vi "Simple F-70 controller.vi"() -> ()   [LabVIEW 2021, in "F-70 controller.lvlib"]
uses:
  F-70 controller.lvlib
  controls/F-70 controller states.ctl
  controls/F-70 controller commands.ctl
  controls/Message to F-70 controller.ctl
  controls/F-70 controller properties.ctl
  <instrlib>/F-70 driver/F-70 driver.lvlib
  <instrlib>/F-70 driver/public/F-70 parameters.ctl
panel:
  out "Event log":string[](array[string])
  in  "Search btn":bool
  out "F-70 parameters":T1 {"Last updated" format="%<%d/%m/%Y %H:%M:%S>T"; "State of operation" items=["Local Off", "Local On", "Remote Off", "Remote On", "Cold head Run", "Cold head pause", "Fault Off", "Oil Fault Off"]; "Return pressure (PSIG)" scale=0.0..200.0; "Water in Tmp (°C)" scale=0.0..100.0; "Water out Tmp (°C)" scale=0.0..100.0; "He discharge Tmp (°C)" scale=0.0..100.0}
  in  "Start Stop Cold head btn":bool
  in  "Exit app btn":bool
  in  "Update interval (ms)":i32=5000
  in  "error in (no error)":errorcluster
  out "error out":errorcluster
  in  "Start Stop btn":bool
  in  "Connect btn":bool
  in  "VISA resource name":refnum<visa-resource-name>
  # "Simple F-70 controller"
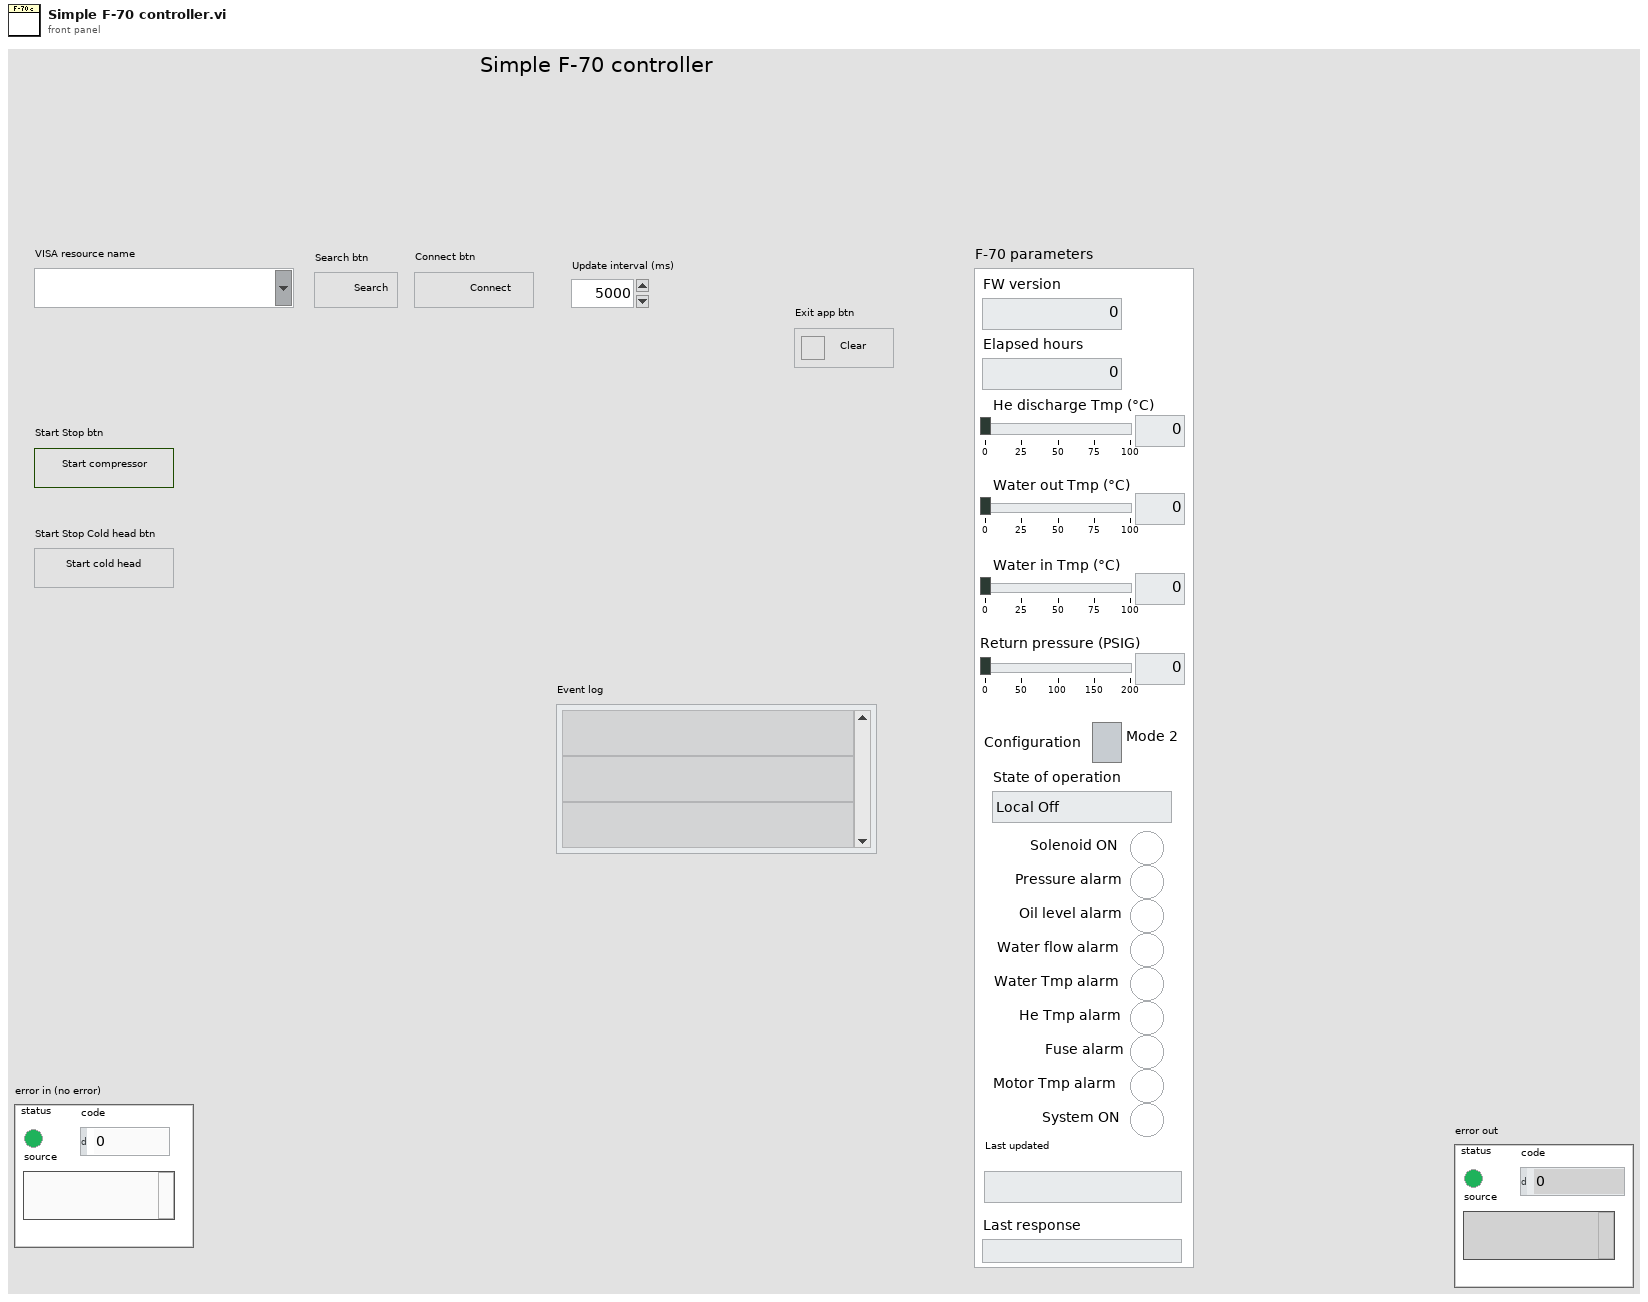
[diagram p1: front panel]
types:
  T1 = typedef "F-70 driver.lvlib/F-70 parameters.ctl" = cluster{"FW version":dbl, "Elapsed hours":dbl, "He discharge Tmp (°C)":dbl, "Water out Tmp (°C)":dbl, "Water in Tmp (°C)":dbl, "Return pressure (PSIG)":dbl, "Configuration":bool, "State of operation":u16, "Solenoid ON":bool, "Pressure alarm":bool, "Oil level alarm":bool, "Water flow alarm":bool, "Water Tmp alarm":bool, "He Tmp alarm":bool, "Fuse alarm":bool, "Motor Tmp alarm":bool, "System ON":bool, "Last updated":timestamp, "Last response":string}
  T2 = typedef "F-70 controller properties.ctl" = cluster{"Connected":bool, "Command msg":T3, "Data msg":variant, "Waiting msgs":i32, "Timeout counter":i32, "Logs":string[]}
  T3 = typedef "F-70 controller commands.ctl" = enum16{"Ignore", "Connect", "Read temperatures", "Read pressure", "Read status", "Update all", "Start compressor", "Stop compressor", "Clear error", "Disconnect"}
  T4 = typedef "F-70 controller.lvlib/F-70 controller states.ctl" = enum16{"Initialize GUI", "Wait for event", "Check message", "Execute command", "Send response", "Sleep", "Search device", "Reserved2", "End"}
  T5 = enum8{"Enabled", "Disabled", "Disabled and Grayed Out"}
  T6 = typedef "Message to F-70 controller.ctl" = cluster{"Command msg":T3, "Data msg":variant}
  T7 = enum16{"Left Button", "Center Button", "Right Button", "Window Close"}
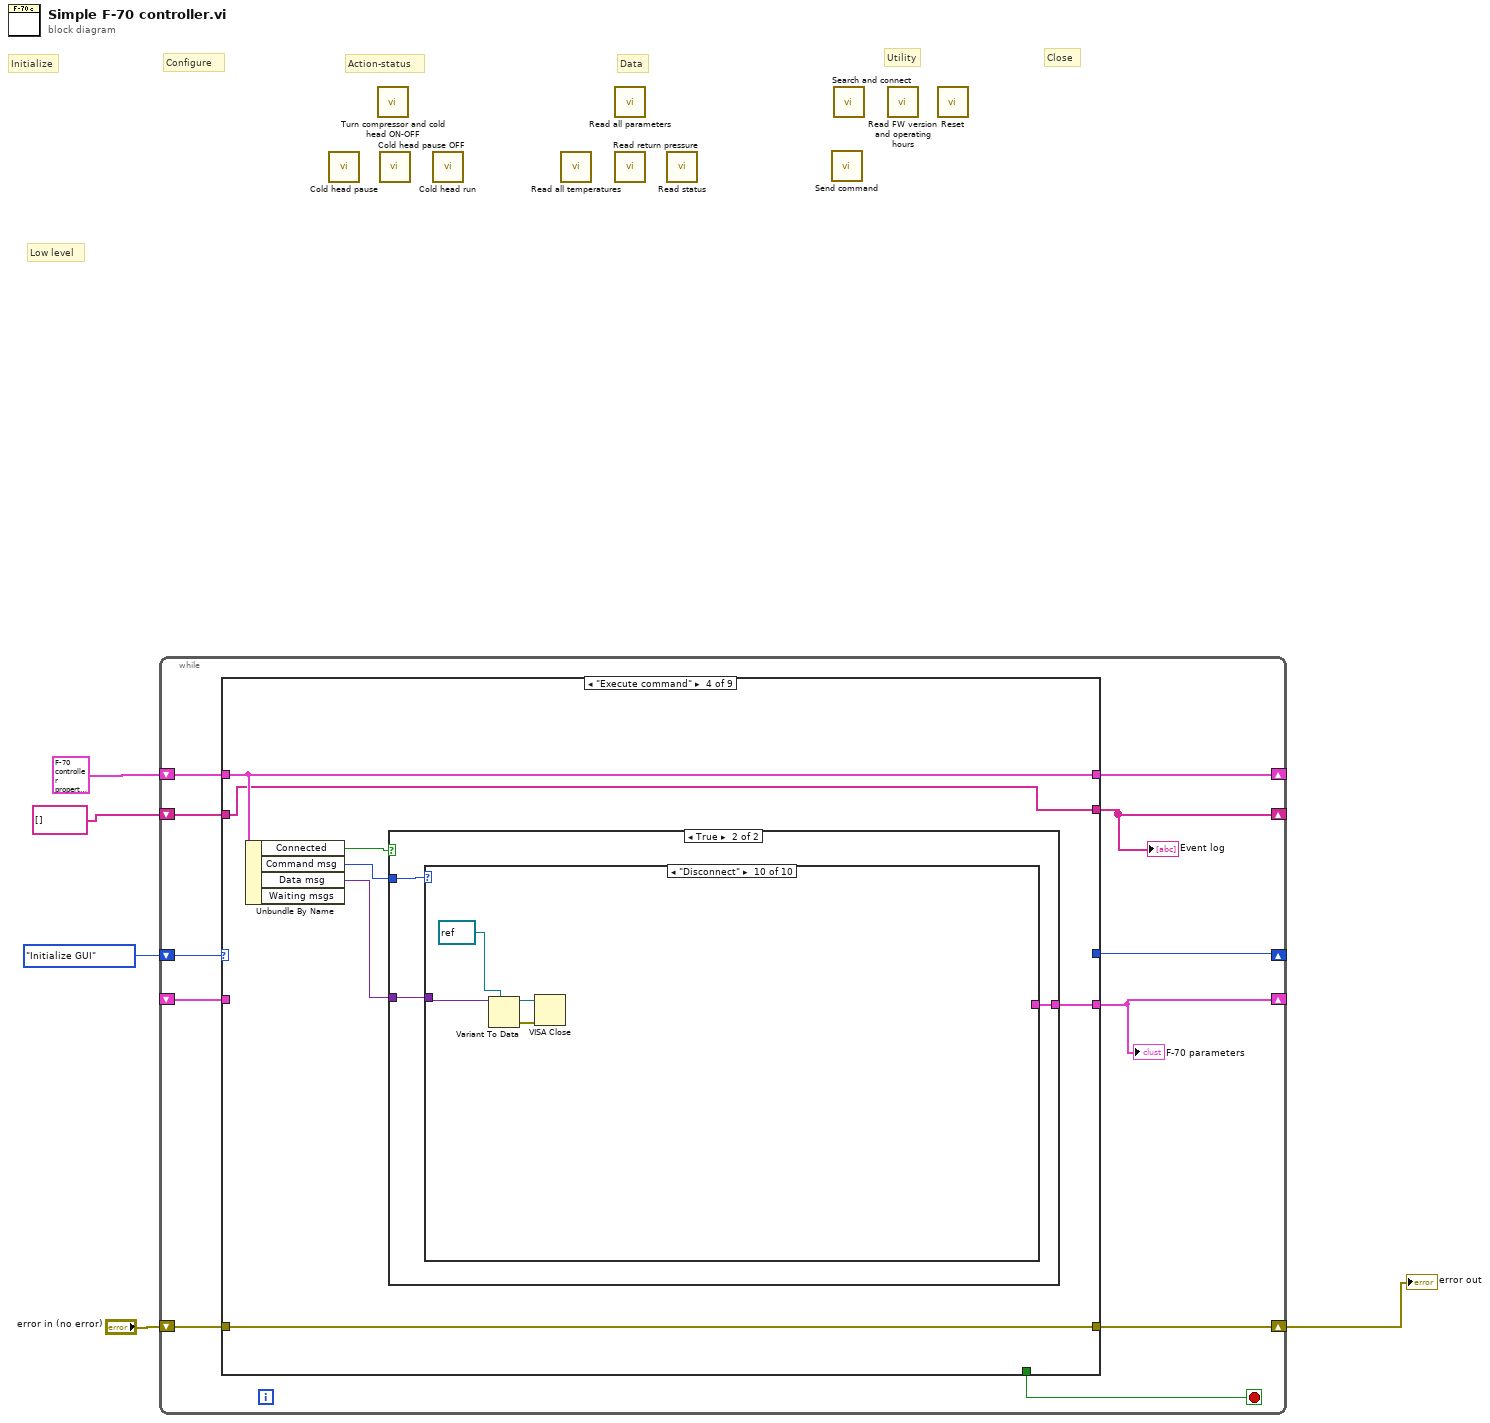
[diagram p0: block diagram]
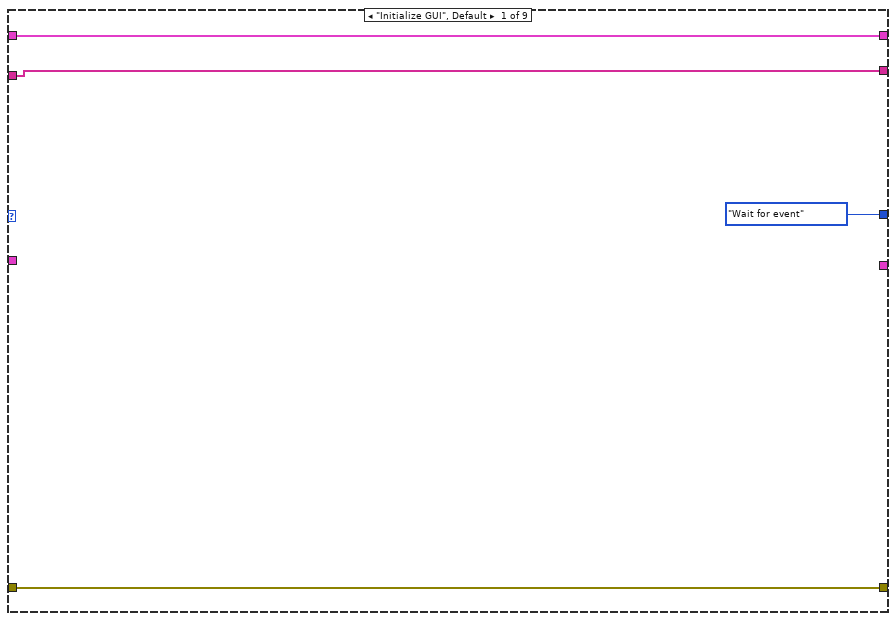
[diagram p2: hidden frame]
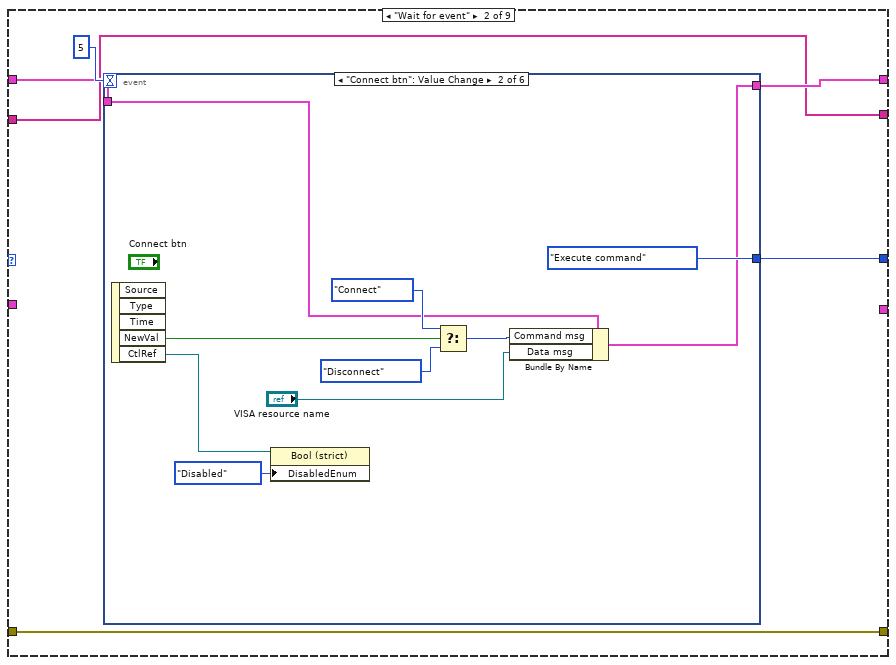
[diagram p3: hidden frame]
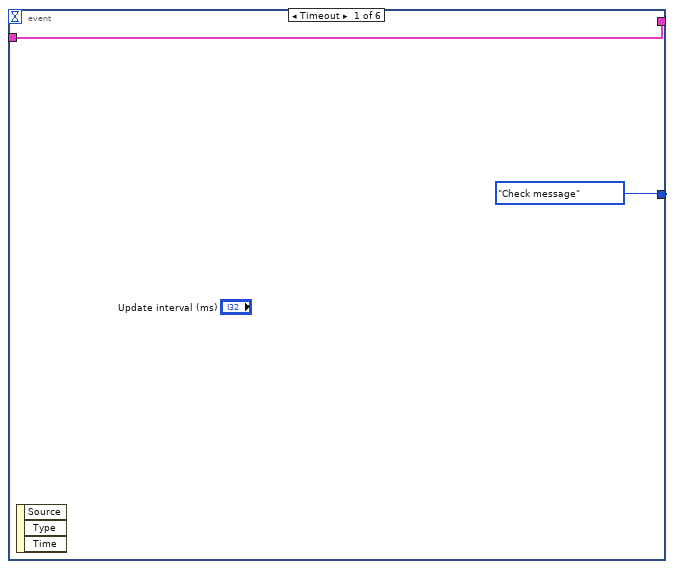
[diagram p4: hidden frame]
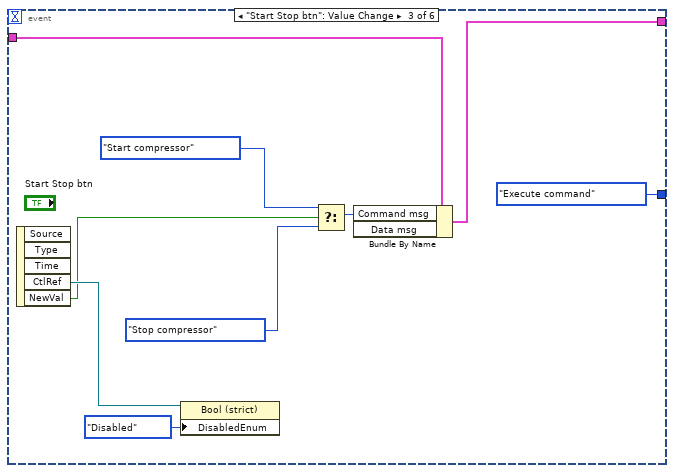
[diagram p5: hidden frame]
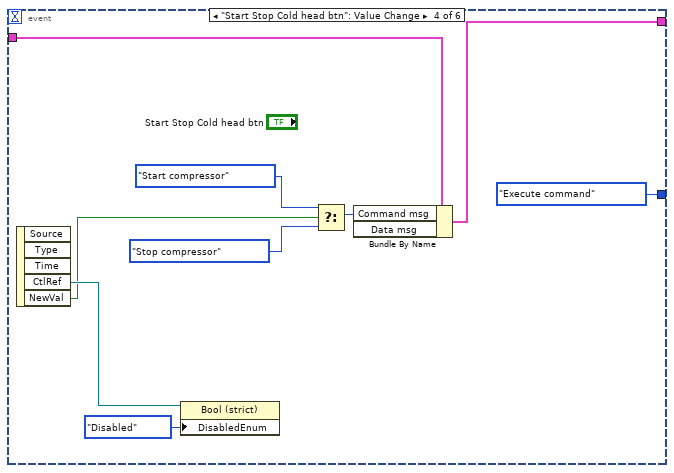
[diagram p6: hidden frame]
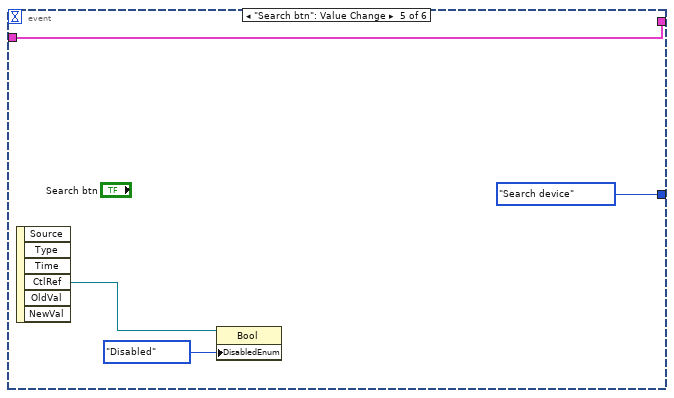
[diagram p7: hidden frame]
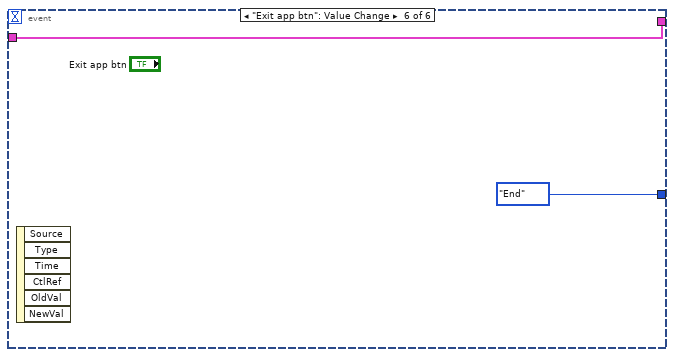
[diagram p8: hidden frame]
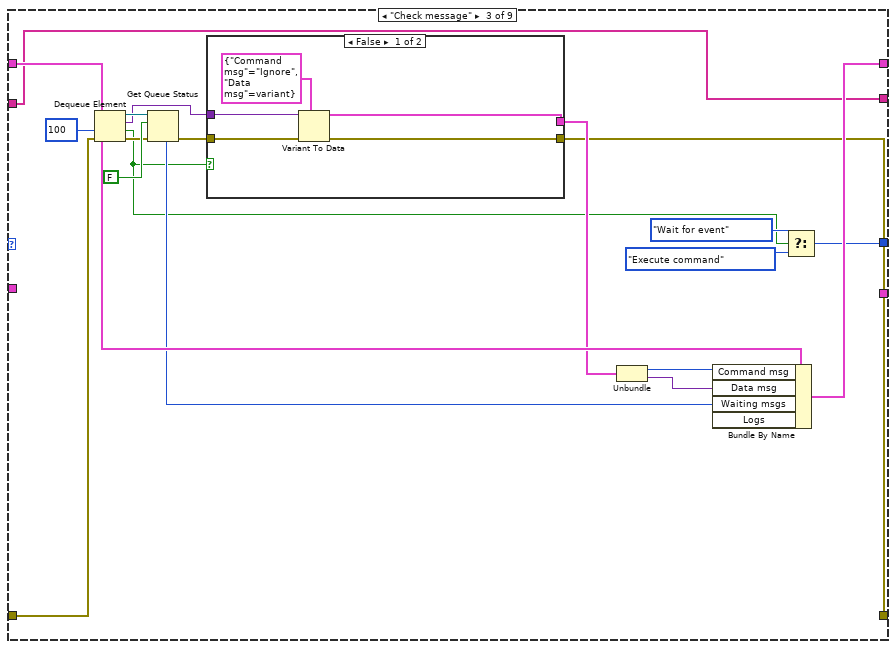
[diagram p9: hidden frame]
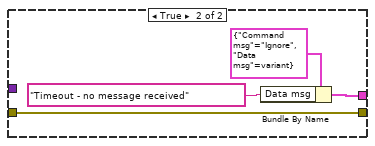
[diagram p10: hidden frame]
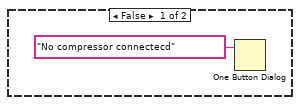
[diagram p11: hidden frame]
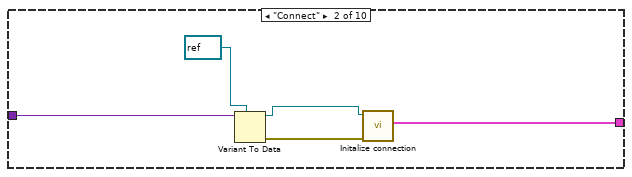
[diagram p13: hidden frame]
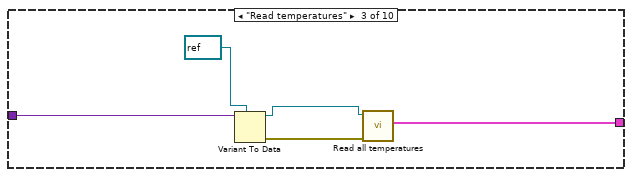
[diagram p14: hidden frame]
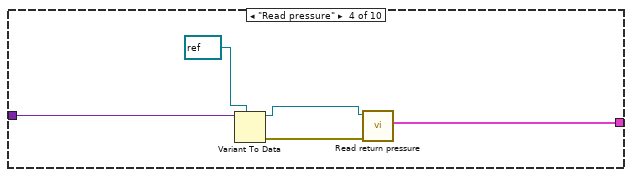
[diagram p15: hidden frame]
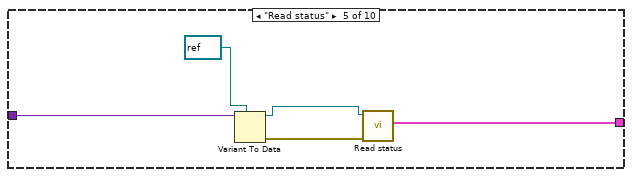
[diagram p16: hidden frame]
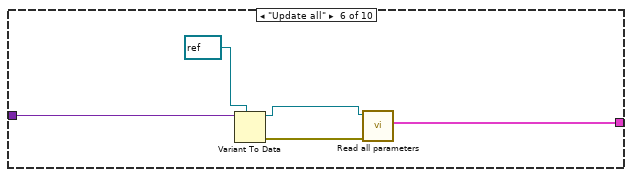
[diagram p17: hidden frame]
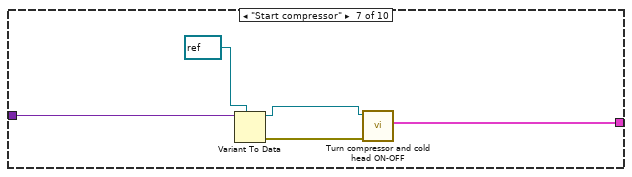
[diagram p18: hidden frame]
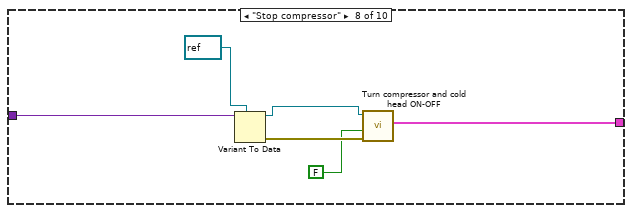
[diagram p19: hidden frame]
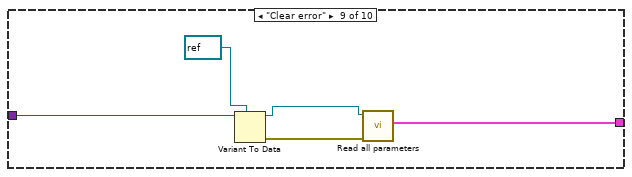
[diagram p20: hidden frame]
diagram:
  # "Low level"
  # "Action-status"
  # "Close"
  # "Utility"
  # "Data"
  # "Configure"
  # "Initialize"
  n1 = while {
    shift-right: [w15] -> _
    shift-left: F-70_controller_states."Initialize GUI" -> [w16]
    shift-right: [w13] -> _
    shift-left: T2 {"Connected"=FALSE, "Command msg"=enum."Ignore", "Data msg"=variant, "Waiting msgs"=0, "Timeout counter"=0, "Logs"=[]} ("F-70 controller properties") -> [w14]
    shift-right: [w11] -> w2
    shift-left: "error in (no error)" -> [w12]
    shift-right: [w10] -> _
    shift-left: string[] [] ("Event log") -> [w9]
    shift-right: [w7] -> _
    shift-left: _ -> [w6]
    stop <- w8 stop-if-true
    n2 = case shown="\"Execute command\"" w16 {
      tunnel: [F-70_controller_states."Wait for event" w25 w67 _ _ _ F-70_controller_states."Wait for event" ("f") _ w165] -> w15
      tunnel: w14 -> [w19 w24 w76 w96 w149 w152 w161 w164 w168]
      tunnel: [w19 w23 w70 w96 w149 w152 w161 w164 w168] -> w13
      tunnel: w12 -> [w18 w22 w77 w97 w148 w151 w160 w163 w170]
      tunnel: [w18 w22 w68 w97 w148 w151 w158 w163 w170] -> w11
      tunnel: w9 -> [w17 w21 w63 w95 w147 w150 w156 w162 w169]
      tunnel: [w17 w21 w63 w95 w147 w150 w156 w162 w169] -> w10
      tunnel: [_ _ _ _ _ _ _ _ w166] -> w8
      tunnel: [_ _ _ w91 _ _ _ _ _] -> w7
      tunnel: w6 -> [_ _ _ _ _ _ _ _ _]
      frame "Initialize GUI", Default {
      }
      frame "Wait for event" {
        n3 = event shown="[1] \"Connect btn\": Value Change" {
          selector: _ -> [_ _ _ _ _ _]
          dyn-events: _ -> [_ _ _ _ _ _]
          timeout: 5 -> [_ _ _ _ _ _]
          tunnel: [F-70_controller_states."Check message" F-70_controller_states."Execute command" F-70_controller_states."Execute command" F-70_controller_states."Execute command" F-70_controller_states."Search device" F-70_controller_states."End"] -> w25
          tunnel: w24 -> [w27 w32 w46 w55 w59 w61]
          tunnel: [w27 w37 w39 w48 w59 w61] -> w23
          event Timeout {
            n4 = event-data() -> ()  [unwired: 1 in, 3 out]
          }
          event "Connect btn": Value Change {
            n5 = event-data() -> ("NewVal"=w34:bool, "CtlRef"=w30:refnum<vi>)  [unwired: 1 in, 3 out]
            n6 = property class="Bool (strict)"(reference=w30, "DisabledEnum"=T5."Disabled" ("Disabled")) -> ()  [unwired: 1 in, 2 out]
            n7 = Select(t=F-70_controller_commands."Connect" ("Command msg"), s=w34, f=F-70_controller_commands."Disconnect") -> (s? t:f=w36:T3)
            n8 = Bundle By Name(cluster=w32, "Command msg"=w36, "Data msg"="VISA resource name") -> (w37:T2)
          }
          event "Start Stop btn": Value Change {
            n9 = event-data() -> ("CtlRef"=w44:refnum<vi>, "NewVal"=w41:bool)  [unwired: 1 in, 3 out]
            n10 = property class="Bool (strict)"(reference=w44, "DisabledEnum"=T5."Disabled" ("Disabled")) -> ()  [unwired: 1 in, 2 out]
            n11 = Select(t=F-70_controller_commands."Start compressor", s=w41, f=F-70_controller_commands."Stop compressor" ("Command msg")) -> (s? t:f=w45:T3)
            n12 = Bundle By Name(cluster=w46, "Command msg"=w45) -> (w39:T2)  [unwired: 1 in]
          }
          event "Start Stop Cold head btn": Value Change {
            n13 = event-data() -> ("CtlRef"=w53:refnum<vi>, "NewVal"=w50:bool)  [unwired: 1 in, 3 out]
            n14 = property class="Bool (strict)"(reference=w53, "DisabledEnum"=T5."Disabled" ("Disabled")) -> ()  [unwired: 1 in, 2 out]
            n15 = Select(t=F-70_controller_commands."Start compressor", s=w50, f=F-70_controller_commands."Stop compressor" ("Command msg")) -> (s? t:f=w54:T3)
            n16 = Bundle By Name(cluster=w55, "Command msg"=w54) -> (w48:T2)  [unwired: 1 in]
          }
          event "Search btn": Value Change {
            n17 = event-data() -> ("CtlRef"=w58:refnum<vi>)  [unwired: 1 in, 5 out]
            n18 = property class="Bool"(reference=w58, "DisabledEnum"=T5."Disabled" ("Disabled")) -> ()  [unwired: 1 in, 2 out]
          }
          event "Exit app btn": Value Change {
            n19 = event-data() -> ()  [unwired: 1 in, 6 out]
          }
        }
      }
      frame "Check message" {
        n20 = Dequeue Element(timeout in ms (-1)=100, error in (no error)=w77) -> (queue out=w78:refnum<queue>, element=w75:variant, timed out?=w65:bool, error out=w79:errorcluster)  [unwired: 1 in]
        n21 = Get Queue Status(queue=w78, return elements? (F)=FALSE, error in (no error)=w79) -> (error out=w74:errorcluster, # elements in queue=w69:i32)  [unwired: 6 out]
        n22 = case shown="False" w65 {
          tunnel: w75 -> [w86 _]
          tunnel: w74 -> [w84 w90]
          tunnel: [w83 w88] -> w73
          tunnel: [w82 w90] -> w68
          frame False {
            n23 = Variant To Data(error in=w84, type=T6 {"Command msg"=enum."Ignore", "Data msg"=variant}, Variant=w86) -> (data=w83:T6, error out=w82:errorcluster)
          }
          frame True {
            n24 = Bundle By Name(cluster=T6 {"Command msg"=enum."Ignore", "Data msg"=variant}, "Data msg"="Timeout - no message received") -> (w88:T6)
          }
        }
        n25 = Unbundle(w73) -> ("Command msg"=w71:T3, "Data msg"=w72:variant)
        n26 = Bundle By Name(cluster=w76, "Command msg"=w71, "Data msg"=w72, "Waiting msgs"=w69) -> (w70:T2)  [unwired: 1 in]
        n27 = Select(t=F-70_controller_states."Wait for event", s=w65, f=F-70_controller_states."Execute command") -> (s? t:f=w67:T4)
      }
      frame "Execute command" {
        n28 = Unbundle By Name(w96) -> ("Connected"=w94:bool, "Command msg"=w93:T3, "Data msg"=w92:variant)  [unwired: 1 out]
        n29 = case shown="True" w94 {
          tunnel: w93 -> [_ w101]
          tunnel: w92 -> [_ w100]
          tunnel: [_ w99] -> w91
          frame False {
            n30 = One Button Dialog(message="No compressor connectecd") -> ()  [unwired: 1 in, 1 out]
          }
          frame True {
            n31 = case shown="\"Disconnect\"" w101 {
              tunnel: w100 -> [_ w103 w108 w113 w118 w123 w128 w134 w139 w143]
              tunnel: [_ w102 w107 w112 w117 w122 w127 w133 w138 _] -> w99
              frame "Ignore", Default {
              }
              frame "Connect" {
                n32 = Variant To Data(type=refnum<visa-resource-name> refnum ("VISA resource name"), Variant=w103) -> (data=w105:refnum<visa-resource-name>, error out=w104:errorcluster)  [unwired: 1 in]
                n33 = call <instrlib>:"Initalize connection.vi"("error in (no error)"=w104, "VISA resource in"=w105) -> ("F-70 parameters out"=w102:T1)  [unwired: 3 in, 2 out]
              }
              frame "Read temperatures" {
                n34 = Variant To Data(type=refnum<visa-resource-name> refnum ("VISA resource name"), Variant=w108) -> (data=w110:refnum<visa-resource-name>, error out=w109:errorcluster)  [unwired: 1 in]
                n35 = call <instrlib>:"Read all temperatures.vi"("error in"=w109, "VISA resource in"=w110) -> ("F-70 parameters out"=w107:T1)  [unwired: 4 in, 5 out]
              }
              frame "Read pressure" {
                n36 = Variant To Data(type=refnum<visa-resource-name> refnum ("VISA resource name"), Variant=w113) -> (data=w115:refnum<visa-resource-name>, error out=w114:errorcluster)  [unwired: 1 in]
                n37 = call <instrlib>:"Read return pressure.vi"("error in"=w114, "VISA resource in"=w115) -> ("F-70 parameters out"=w112:T1)  [unwired: 2 in, 3 out]
              }
              frame "Read status" {
                n38 = Variant To Data(type=refnum<visa-resource-name> refnum ("VISA resource name"), Variant=w118) -> (data=w120:refnum<visa-resource-name>, error out=w119:errorcluster)  [unwired: 1 in]
                n39 = call <instrlib>:"Read status.vi"("error in"=w119, "VISA resource in"=w120) -> ("F-70 parameters out"=w117:T1)  [unwired: 2 in, 3 out]
              }
              frame "Update all" {
                n40 = Variant To Data(type=refnum<visa-resource-name> refnum ("VISA resource name"), Variant=w123) -> (data=w125:refnum<visa-resource-name>, error out=w124:errorcluster)  [unwired: 1 in]
                n41 = call <instrlib>:"Read all parameters.vi"("error in"=w124, "VISA resource in"=w125) -> ("F-70 parameters out"=w122:T1)  [unwired: 3 in, 2 out]
              }
              frame "Start compressor" {
                n42 = Variant To Data(type=refnum<visa-resource-name> refnum ("VISA resource name"), Variant=w128) -> (data=w130:refnum<visa-resource-name>, error out=w129:errorcluster)  [unwired: 1 in]
                n43 = call <instrlib>:"Turn compressor and cold head ON-OFF.vi"("error in"=w129, "VISA resource in"=w130) -> ("F-70 parameters out"=w127:T1)  [unwired: 6 in, 3 out]
              }
              frame "Stop compressor" {
                n44 = Variant To Data(type=refnum<visa-resource-name> refnum ("VISA resource name"), Variant=w134) -> (data=w136:refnum<visa-resource-name>, error out=w135:errorcluster)  [unwired: 1 in]
                n45 = call <instrlib>:"Turn compressor and cold head ON-OFF.vi"("error in"=w135, "Action (ON)"=FALSE, "VISA resource in"=w136) -> ("F-70 parameters out"=w133:T1)  [unwired: 5 in, 3 out]
              }
              frame "Clear error" {
                n46 = Variant To Data(type=refnum<visa-resource-name> refnum ("VISA resource name"), Variant=w139) -> (data=w141:refnum<visa-resource-name>, error out=w140:errorcluster)  [unwired: 1 in]
                n47 = call <instrlib>:"Read all parameters.vi"("error in"=w140, "VISA resource in"=w141) -> ("F-70 parameters out"=w138:T1)  [unwired: 3 in, 2 out]
              }
              frame "Disconnect" {
                n48 = Variant To Data(type=refnum<visa-resource-name> refnum ("VISA resource name"), Variant=w143) -> (data=w145:refnum<visa-resource-name>, error out=w144:errorcluster)  [unwired: 1 in]
                n49 = VISA Close(VISA resource name=w145, error in (no error)=w144) -> ()  [unwired: 1 out]
              }
            }
          }
        }
      }
      frame "Send response" {
      }
      frame "Sleep" {
      }
      frame "Search device" {
        n50 = call <instrlib>:"Search and connect.vi"("error in"=w160) -> ("error out"=w154:errorcluster, "VISA resource out"=w155:refnum<visa-resource-name>)  [unwired: 9 in]
        n51 = call <vilib>:"Simple Error Handler.vi"("error in (no error)"=w154) -> ("error out"=w153:errorcluster)  [unwired: 4 in, 4 out]
        n52 = local write "VISA resource name"(w155) -> ()
        n53 = VISA Close(VISA resource name=w155, error in (no error)=w153) -> (error out=w158:errorcluster)
        n54 = property on="Search btn" class="Bool"(error in=w158, "DisabledEnum"=T5."Disabled" ("Disabled")) -> ()  [unwired: 1 in, 2 out]
      }
      frame "Reserved2" {
      }
      frame "End" {
        n55 = Unbundle By Name(w168) -> ("Connected"=w167:bool)
        n56 = case shown="True" w167 {
          tunnel: [TRUE w173] -> w166
          tunnel: [_ w172] -> w165
          frame False {
          }
          frame True {
            n57 = call <vilib>:"Three Button Dialog.vi"("message"="Compressor is still connected.\nDo you want to disconnect it\nbefore exit?") -> ("Which Button?"=w174:T7)  [unwired: 10 in]
            n58 = case shown="\"Center Button\"" w174 {
              tunnel: [TRUE TRUE TRUE] -> w173
              tunnel: [_ _ F-70_controller_states."Wait for event" ("f")] -> w172
              frame "Left Button", Default {
                n59 = local read "VISA resource name"() -> (w176:refnum<visa-resource-name>)
                n60 = VISA Close(VISA resource name=w176) -> ()  [unwired: 1 in, 1 out]
              }
              frame "Center Button" {
              }
              frame "Right Button" {
              }
            }
          }
        }
      }
    }
    "Event log" <- w10
    "F-70 parameters" <- w7
  }
  "error out" <- w2
  n61 = call <instrlib>:"Cold head pause.vi"() -> ()  [unwired: 8 in, 4 out]
  n62 = call <instrlib>:"Turn compressor and cold head ON-OFF.vi"() -> ()  [unwired: 8 in, 4 out]
  n63 = call <instrlib>:"Cold head pause OFF.vi"() -> ()  [unwired: 8 in, 4 out]
  n64 = call <instrlib>:"Cold head run.vi"() -> ()  [unwired: 8 in, 4 out]
  n65 = call <instrlib>:"Read all temperatures.vi"() -> ()  [unwired: 6 in, 6 out]
  n66 = call <instrlib>:"Read all parameters.vi"() -> ()  [unwired: 5 in, 3 out]
  n67 = call <instrlib>:"Read return pressure.vi"() -> ()  [unwired: 4 in, 4 out]
  n68 = call <instrlib>:"Read status.vi"() -> ()  [unwired: 4 in, 4 out]
  n69 = call <instrlib>:"Send command.vi"() -> ()  [unwired: 5 in, 3 out]
  n70 = call <instrlib>:"Search and connect.vi"() -> ()  [unwired: 10 in, 2 out]
  n71 = call <instrlib>:"Read FW version and operating hours.vi"() -> ()  [unwired: 7 in, 5 out]
  n72 = call <instrlib>:"Reset.vi"() -> ()  [unwired: 9 in, 3 out]
